vi "end_laser_q.vi"(7 "Laser Power Q In":T1) -> (15 "error out":errorcluster)   [LabVIEW 2023]
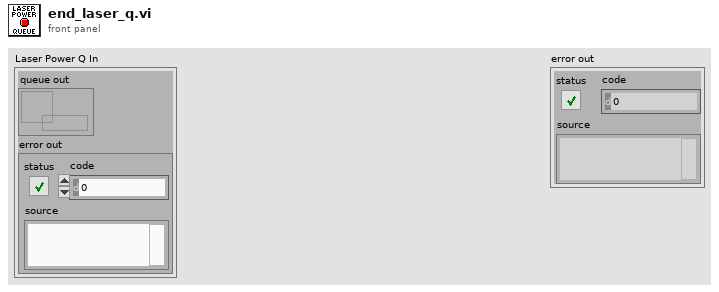
[diagram p1: front panel]
types:
  T1 = cluster{"queue out":refnum<queue>, "error out":errorcluster}
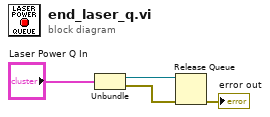
[diagram p0: block diagram]
diagram:
  n1 = Unbundle("Laser Power Q In") -> ("queue out"=w3:refnum<queue>, "error out"=w2:errorcluster)
  n2 = Release Queue(queue=w3, error in (no error)=w2) -> (error out=→"error out":errorcluster)  [unwired: 1 in, 2 out]
